vi "findBlinkTimeLIA.vi"(1 "refarr":T1, 2 "maxperiod":i32=4) -> (0 "adjustedperiod":i32)   [LabVIEW 2017]
uses:
  RefArray/RefArray.ctl
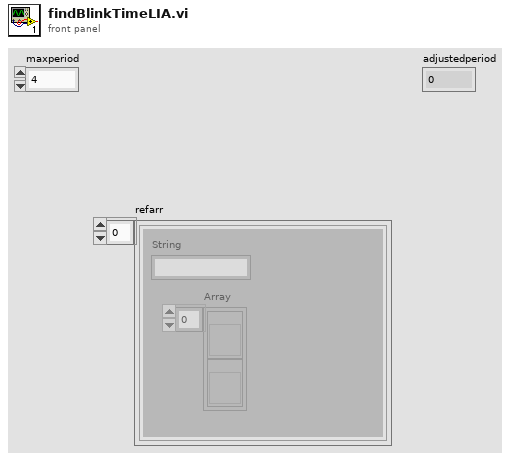
[diagram p1: front panel]
types:
  T1 = typedef "RefArray.ctl" = cluster{"String":string, "Array":refnum<vi>[]}[]
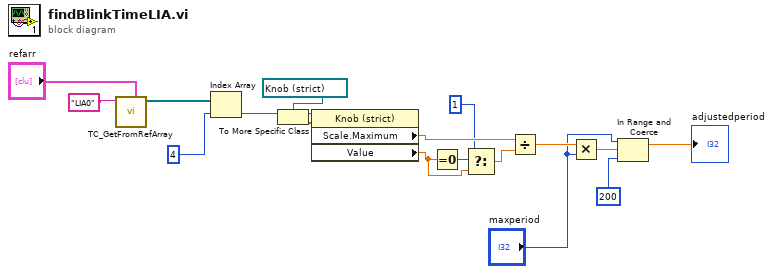
[diagram p0: block diagram]
diagram:
  n1 = call "TC_GetFromRefArray.vi"("arrayIn"="refarr", "NameToFind"="LIA0") -> ("refArray"=w16:refnum<vi>[])  [unwired: 8 in, 1 out]
  n2 = Index Array(array=w16, index=4) -> (element=w14:refnum<vi>)
  n3 = To More Specific Class(target class=refnum<vi> refnum ("Chopping Frequency"), reference=w14) -> (specific class reference=w13:refnum<vi>, error out=w12:errorcluster)  [unwired: 1 in]
  n4 = property class="Knob (strict)"(reference=w13, error in=w12) -> ("Scale.Maximum"=w10:dbl, "Value"=w8:dbl)  [unwired: 2 out]
  n5 = Equal To 0?(x=w8) -> (x = 0?=w9:bool)
  n6 = Select(t=1, s=w9, f=w8) -> (s? t:f=w6:dbl)
  n7 = Divide(x=w10, y=w6) -> (x/y=w2:dbl)
  n8 = Multiply(x=w2, y="maxperiod") -> (x*y=w5:dbl)
  n9 = In Range and Coerce(upper limit="maxperiod", x=w5, lower limit=200) -> (coerced(x)=→"adjustedperiod":dbl)  [unwired: 1 out]
